vi "LabJackT7-Silos.vi"(4 "Scan Period":dbl format="%.2f", 5 "Previous Scan Value":dbl format="%.2f", 6 "Present scan array":dbl[](array[numeric]) format="%.2f", 7 "Value to Output":dbl format="%.2f", 8 "Ch Description":T1={"Ch Name"="", "Type"="", "Function"=enum."Analogue Input", "Ch State"=enum."On", "Calibration type"=enum."Raw", "A"=0.0, "B"=0.0, "C"=0.0, "D"=0.0, "Comments"="", "Address"={"Main"=0, "Ch."=0, "Sub"=0, "Port Name"=""}, "String"="", "Duty"=65535} {"Duty" format="%.0b"; "D" format="%#_5g"; "C" format="%#_5g"; "B" format="%#_5g"; "A" format="%#_5g"}, 9 "Ch names":string[](array[string])) -> (0 "Scan comment":string, 1 "Output":dbl format="%.7f")   [LabVIEW 2015]
uses:
  ADAM Client/Sub VIs/ADAM Controls/Ch_description_ADAM.ctl
  ADAM Client/Sub VIs/ADAM Controls/Module_type_ADAM.ctl
  ADAM Client/Sub VIs/ADAM Controls/Function_ADAM.ctl
  ADAM Client/Sub VIs/ADAM Controls/Channel_State.ctl
  ADAM Client/Sub VIs/ADAM Controls/Calib_type_ADAM.ctl
  ADAM Client/Sub VIs/ADAM Controls/Address.ctl
  ADAM Client/Sub VIs/ADAM Controls/Remember_value_mode.ctl
  <vilib>/Utility/error.llb/DialogType.ctl
panel:
  in  "Value to Output 2":dbl format="%.2f"
  out "t2":dbl
  out "t1":dbl
  out "elapsed t (sec)":dbl
  in  "MaxAge(s)":dbl=1.5
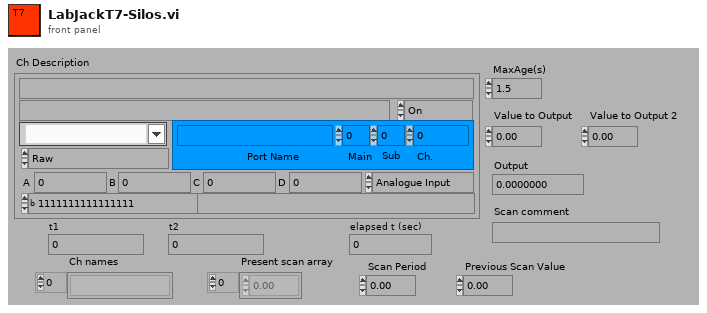
[diagram p1: front panel]
types:
  T1 = typedef "Ch_description_ADAM.ctl" = cluster{"Ch Name":string, "Type":T2, "Function":T3, "Ch State":T4, "Calibration type":T5, "A":dbl, "B":dbl, "C":dbl, "D":dbl, "Comments":string, "Address":T6, "String":string, "Duty":u16}
  T2 = typedef "Module_type_ADAM.ctl" = string
  T3 = typedef "Function_ADAM.ctl" = enum16{"Analogue Input", "Digital Input", "Event counter", "Event rate", "Analogue Output", "Digital Output", "Relay Output"}
  T4 = typedef "Channel_State.ctl" = enum16{"On", "Off", "Always On", "Always Off"}
  T5 = typedef "Calib_type_ADAM.ctl" = enum16{"Raw", "Bx + A", "Cx^2 + Bx + A", "Dx^3 + Cx^2 + Bx + A", "In Band", "Hi-Tec Q", "Hi-Tec M_dot", "Text"}
  T6 = typedef "Address.ctl" = cluster{"Main":i32, "Ch.":i32, "Sub":i32, "Port Name":string}
  T7 = typedef "Remember_value_mode.ctl" = enum16{"Read only", "Read and Write"}
  T8 = typedef "DialogType.ctl" = u16
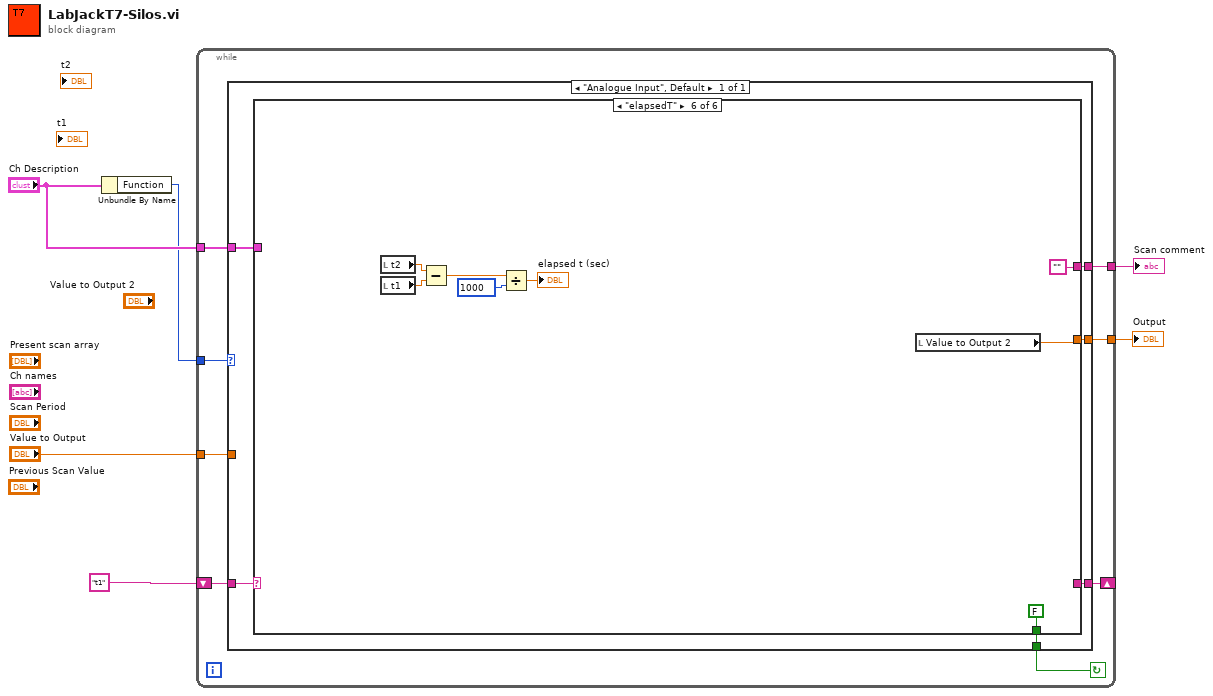
[diagram p0: block diagram]
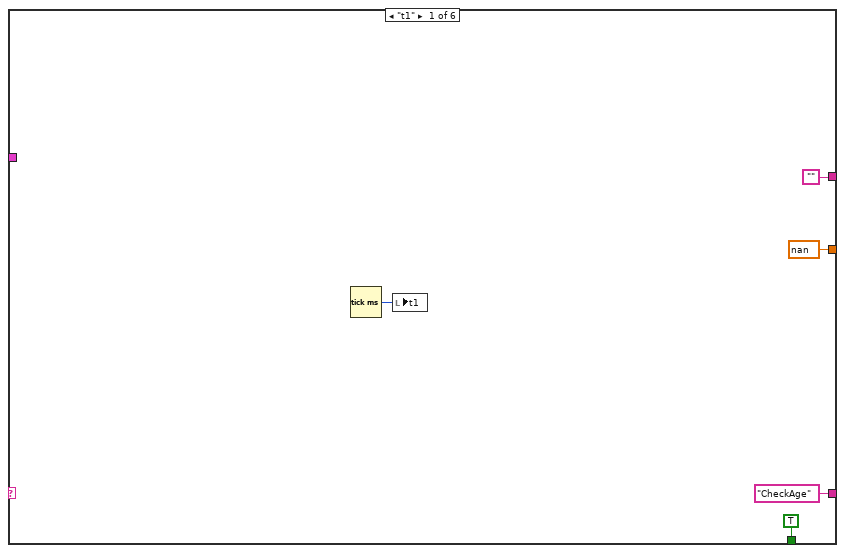
[diagram p2: hidden frame]
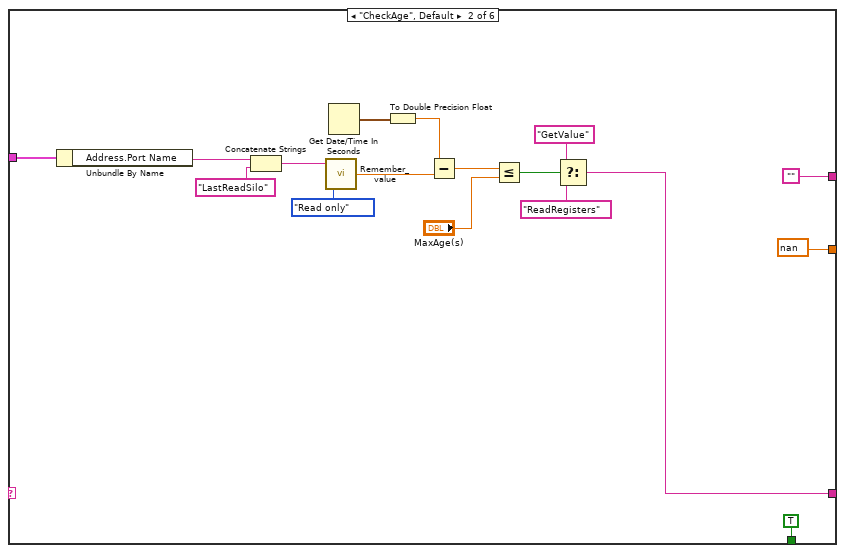
[diagram p3: hidden frame]
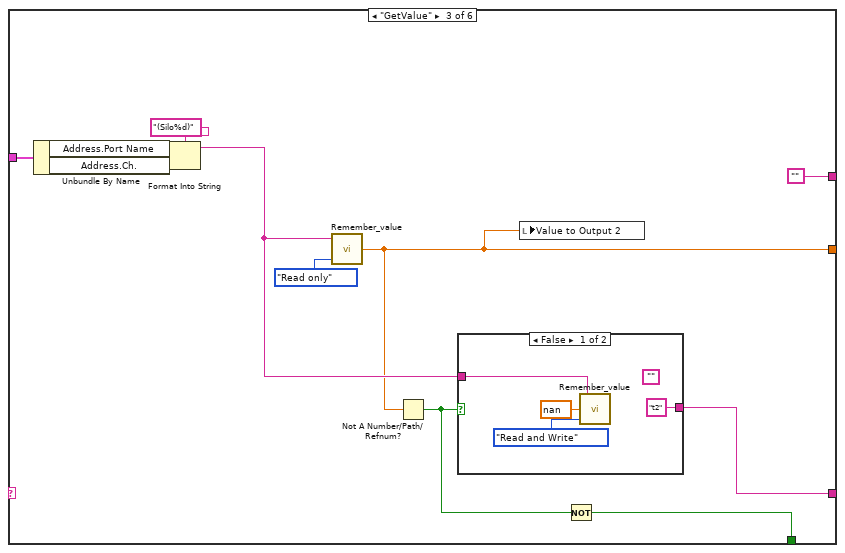
[diagram p4: hidden frame]
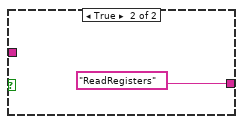
[diagram p5: hidden frame]
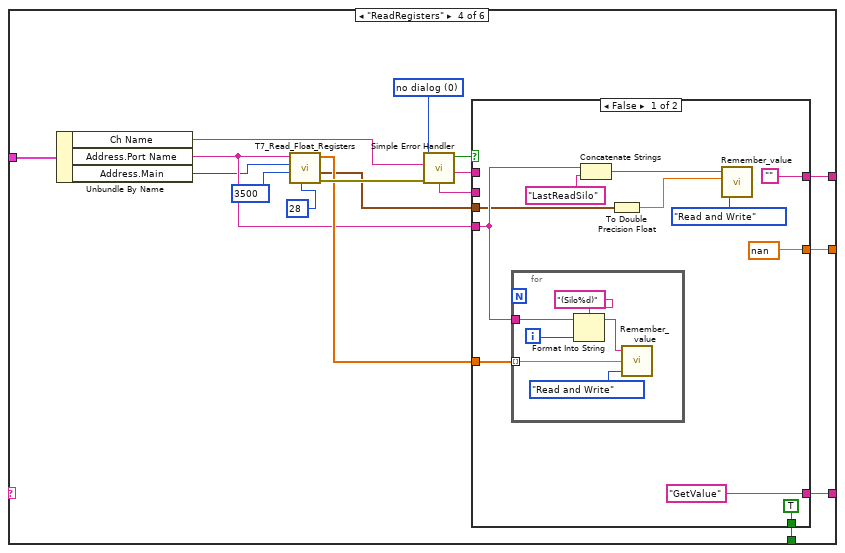
[diagram p6: hidden frame]
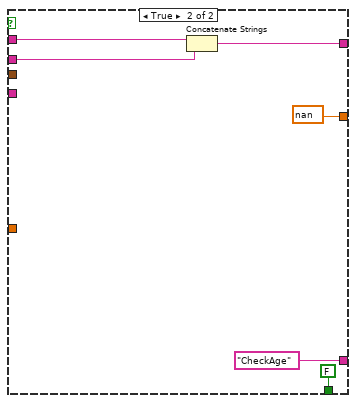
[diagram p7: hidden frame]
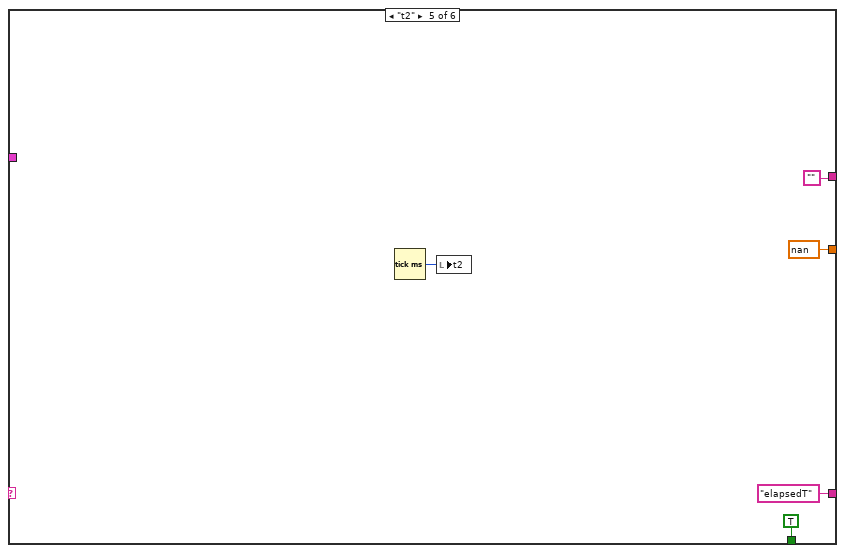
[diagram p8: hidden frame]
diagram:
  n1 = Unbundle By Name("Ch Description") -> ("Function"=w2:T3)
  n2 = while {
    tunnel: "Ch Description" -> [w14]
    tunnel: [w13] -> w6
    shift-right: [w11] -> _
    shift-left: "t1" -> [w12]
    tunnel: [w9] -> w4
    tunnel: w2 -> [w8]
    tunnel: "Value to Output" -> [w7]
    stop <- w10 continue-if-true
    n3 = case shown="\"Analogue Input\", Default" w8 {
      tunnel: w14 -> [w20]
      tunnel: [w19] -> w13
      tunnel: w12 -> [w18]
      tunnel: [w17] -> w11
      tunnel: [w16] -> w10
      tunnel: [w15] -> w9
      tunnel: w7 -> [_]
      frame "Analogue Input", Default {
        n4 = case shown="\"elapsedT\"" w18 {
          tunnel: w20 -> [_ w39 w53 w75 _ _]
          tunnel: ["" "" "" w69 "" ""] -> w19
          tunnel: ["CheckAge" w29 w47 w63 "elapsedT" _] -> w17
          tunnel: [TRUE TRUE w44 w60 TRUE FALSE] -> w16
          tunnel: [nan ("Output Value") nan w43 w59 nan ("Output Value") w105] -> w15
          frame "t1" {
            n5 = Tick Count (ms)() -> (millisecond timer value=w25:u32)
            n6 = local write "t1"(w25) -> ()
          }
          frame "CheckAge", Default {
            n7 = Unbundle By Name(w39) -> ("Address.Port Name"=w38:string)
            n8 = Concatenate Strings(w38, "LastReadSilo" ("string")) -> (w42:string)
            n9 = call "Remember_value.vi"("Mode"=Remember_value_mode."Read only", "Ch name"=w42) -> ("Output Value"=w35:dbl)  [unwired: 1 in]
            n10 = Get Date/Time In Seconds() -> (seconds since 1Jan1904=w37:timestamp)
            n11 = To Double Precision Float(number=w37) -> (double precision float=w36:dbl)
            n12 = Subtract(x=w36, y=w35) -> (x-y=w34:dbl)
            n13 = Less Or Equal?(x=w34, y="MaxAge(s)") -> (x <= y?=w32:bool)
            n14 = Select(t="GetValue", s=w32, f="ReadRegisters") -> (s? t:f=w29:string)
          }
          frame "GetValue" {
            n15 = Unbundle By Name(w53) -> ("Address.Port Name"=w49:string, "Address.Ch."=w50:i32)
            n16 = Format Into String(format string="(Silo%d)", initial string=w49, w50) -> (resulting string=w45:string)  [unwired: 1 in, 1 out]
            n17 = call "Remember_value.vi"("Mode"=Remember_value_mode."Read only", "Ch name"=w45) -> ("Output Value"=w43:dbl)  [unwired: 1 in]
            n18 = Not A Number/Path/Refnum?(number/path/refnum=w43) -> (NaN/Path/Refnum?=w46:bool)
            n19 = case shown="False" w46 {
              tunnel: ["t2" "ReadRegisters"] -> w47
              tunnel: w45 -> [w56 _]
              frame False {
                (unwired) ""
                n20 = call "Remember_value.vi"("Mode"=Remember_value_mode."Read and Write", "Input Value"=nan, "Ch name"=w56) -> ()  [unwired: 1 out]
              }
              frame True {
              }
            }
            n21 = local write "Value to Output 2"(w43) -> ()
            n22 = Not(x=w46) -> (.not. x?=w44:bool)
          }
          frame "ReadRegisters" {
            w74 = T8 0 items=["no dialog", "OK message", "continue or stop message", "OK message + warnings", "continue/stop + warnings"] ("type of dialog (OK msg:1)")
            n23 = Unbundle By Name(w75) -> ("Ch Name"=w71:string, "Address.Port Name"=w62:string, "Address.Main"=w61:i32)
            n24 = call "T7_Read_Float_Registers.vi"("Num Registers"=u16 28, "FirstChannel"=u16 3500 ("Starting Address"), "Remote Port"=w61, "Remote IP Address"=w62) -> ("error out"=w68:errorcluster, "ReadAt"=w64:timestamp, "Array"=w65:dbl[])  [unwired: 4 in, 1 out]
            n25 = call <vilib>:"Simple Error Handler.vi"("error source (\" \")"=w71, "type of dialog (OK msg:1)"=w74, "error in (no error)"=w68) -> ("error?"=w70:bool, "source out"=w72:string, "message"=w73:string)  [unwired: 4 out]
            n26 = case shown="False" w70 {
              tunnel: w73 -> [_ w97]
              tunnel: w72 -> [_ w98]
              tunnel: ["" w96] -> w69
              tunnel: w62 -> [w82 _]
              tunnel: w65 -> [w81 _]
              tunnel: w64 -> [w80 _]
              tunnel: ["GetValue" "CheckAge"] -> w63
              tunnel: [TRUE FALSE] -> w60
              tunnel: [nan nan] -> w59
              frame False {
                n27 = for {
                  tunnel: w81 -> [w92] mode=indexing
                  tunnel: w82 -> [w91]
                  i -> [w87]
                  n28 = Format Into String(format string="(Silo%d)", initial string=w91, w87) -> (resulting string=w90:string)  [unwired: 1 in, 1 out]
                  n29 = call "Remember_value.vi"("Mode"=Remember_value_mode."Read and Write", "Input Value"=w92, "Ch name"=w90) -> ()  [unwired: 1 out]
                }
                n30 = Concatenate Strings(w82, "LastReadSilo" ("string")) -> (w85:string)
                n31 = To Double Precision Float(number=w80) -> (double precision float=w79:dbl)
                n32 = call "Remember_value.vi"("Mode"=Remember_value_mode."Read and Write", "Input Value"=w79, "Ch name"=w85) -> ()  [unwired: 1 out]
              }
              frame True {
                n33 = Concatenate Strings(w98, w97) -> (w96:string)
              }
            }
          }
          frame "t2" {
            n34 = Tick Count (ms)() -> (millisecond timer value=w103:u32)
            n35 = local write "t2"(w103) -> ()
          }
          frame "elapsedT" {
            n36 = local read "t2"() -> (w111:dbl)
            n37 = local read "t1"() -> (w110:dbl)
            n38 = Subtract(x=w111, y=w110) -> (x-y=w107:dbl)
            n39 = Divide(x=w107, y=u32 1000) -> (x/y=→"elapsed t (sec)":dbl)
            n40 = local read "Value to Output 2"() -> (w105:dbl)
          }
        }
      }
    }
  }
  "Output" <- w4
  "Scan comment" <- w6
